vi "Cal IC (Numeric).vi"(8 "error in (no error)":errorcluster, 10 "IC in":variant, 11 "Domain_Evolut_1D in":refnum<class "NI_Domain_Evolut_1D.lvclass">) -> (0 "error out":errorcluster, 2 "IC out":variant, 3 "Domain_Evolut_1D out":refnum<class "NI_Domain_Evolut_1D.lvclass">)   [LabVIEW 2017, in "NI_PDE.lvlib" / "NI_Domain_Evolut_1D.lvclass"]
uses:
  <vilib>/gmath/pde.llb/DomainClass/Domain_Evolut_1D/NI_Domain_Evolut_1D.lvclass
  <vilib>/gmath/pde.llb/ICClass/IC_1D_Numeric/IC Data.ctl
  <vilib>/gmath/pde.llb/Common/PDE_IC Type.ctl
  <vilib>/gmath/pde.llb/DomainClass/Domain_Evolut_1D/NI_Domain_Evolut_1D.lvclass/NI_Domain_Evolut_1D.ctl
  <vilib>/gmath/NI_PDE.lvlib
  <vilib>/gmath/pde.llb/ICClass/IC_1D_Numeric/NI_IC_1D_Numeric.lvclass
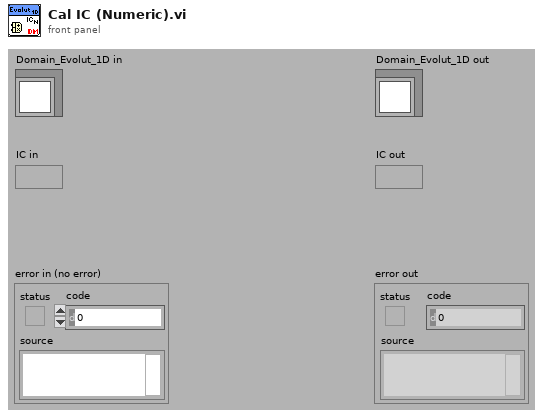
[diagram p1: front panel]
types:
  T1 = typedef "NI_PDE.lvlib/NI_IC_1D_Numeric.lvclass/IC Data.ctl" = cluster{"type":T2, "H":dbl[]}
  T2 = typedef "NI_PDE.lvlib/PDE_IC Type.ctl" = i32
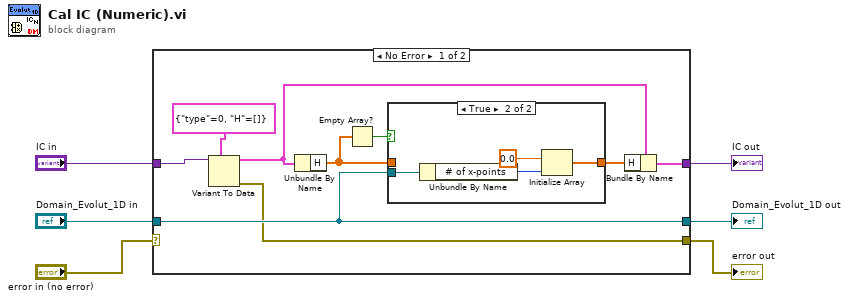
[diagram p0: block diagram]
diagram:
  n1 = case shown="No Error" "error in (no error)" {
    selector: "error in (no error)" -> [_ w23]
    tunnel: "Domain_Evolut_1D in" -> [w8 w22]
    tunnel: [w8 w22] -> w6
    tunnel: [w7 w23] -> w5
    tunnel: [w9 w21] -> w2
    tunnel: "IC in" -> [w14 w21]
    frame No Error {
      n2 = Variant To Data(type=T1 {"type"=0, "H"=[]} ("IC data"), Variant=w14) -> (data=w11:T1, error out=w7:errorcluster)  [unwired: 1 in]
      n3 = Unbundle By Name(w11) -> ("H"=w12:dbl[])
      n4 = Empty Array?(array=w12) -> (empty?=w15:bool)
      n5 = case shown="True" w15 {
        tunnel: w8 -> [_ w18]
        tunnel: w12 -> [w16 _]
        tunnel: [w16 w20] -> w10
        frame False {
        }
        frame True {
          n6 = Unbundle By Name(w18) -> ("# of x-points"=w17:i32)
          n7 = Initialize Array(0.0 ("element"), w17) -> (w20:dbl[])
        }
      }
      n8 = Bundle By Name(cluster=w11, "H"=w10) -> (w9:T1)
    }
    frame Error {
    }
  }
  "Domain_Evolut_1D out" <- w6
  "error out" <- w5
  "IC out" <- w2
